vi "gaussmeter_setup.vi"(0 "VISA resource name Gaussmeter":refnum<visa-resource-name>, 1 "Switch Gaussmeter":bool, 2 "Gaussmeter Number":u8, 3 "Moving Gaussmeter":bool, 4 "x Gaussmeter":dbl, 5 "error in (no error)":errorcluster, 7 "y Gaussmeter":dbl, 9 "z Gaussmeter":dbl) -> (6 "Probe Type":u16(ring)=40 items=["High Sensitivity"=40, "High Stability"=41, "Ultra-High Sensitivity"=42, "User Programmable Cable / High Sensitivity Probe"=50, "User Programmable Cable / High Stability Probe"=51, "User Programmable Cable / Ultra-High Sensitivity Probe"=52], 8 "Probe Serial Number":string, 10 "Probe Sensitivity":dbl=0.001 format="%^.3e", 12 "Probe Field\nCompensation On":bool, 13 "Status Gaussmeter":bool, 14 "Gaussmeter VISA resource name out":refnum<visa-resource-name>, 15 "Field Range":u16(ring)=1 items=["1 - Lowest"=1, "2"=2, "3"=3, "4 - Highest"=4], 16 "Field Units":u16(ring)=1 items=["Gauss"=1, "Tesla"=2, "Oersted"=3, "Amp/Meter"=4], 17 "Auto Range On":bool, 18 "Text Output":string, 19 "error out":errorcluster)   [LabVIEW 2016]
uses:
  <instrlib>/Lake Shore 425/Lake Shore 425.lvlib
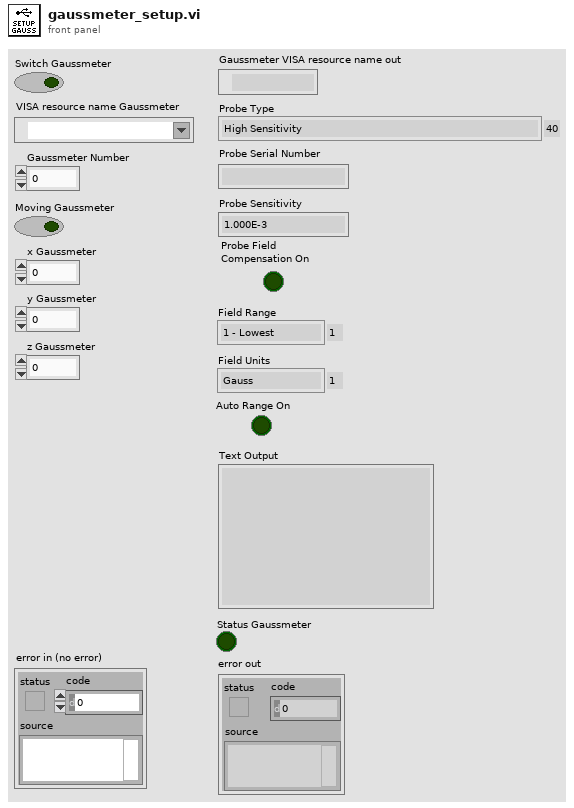
[diagram p1: front panel]
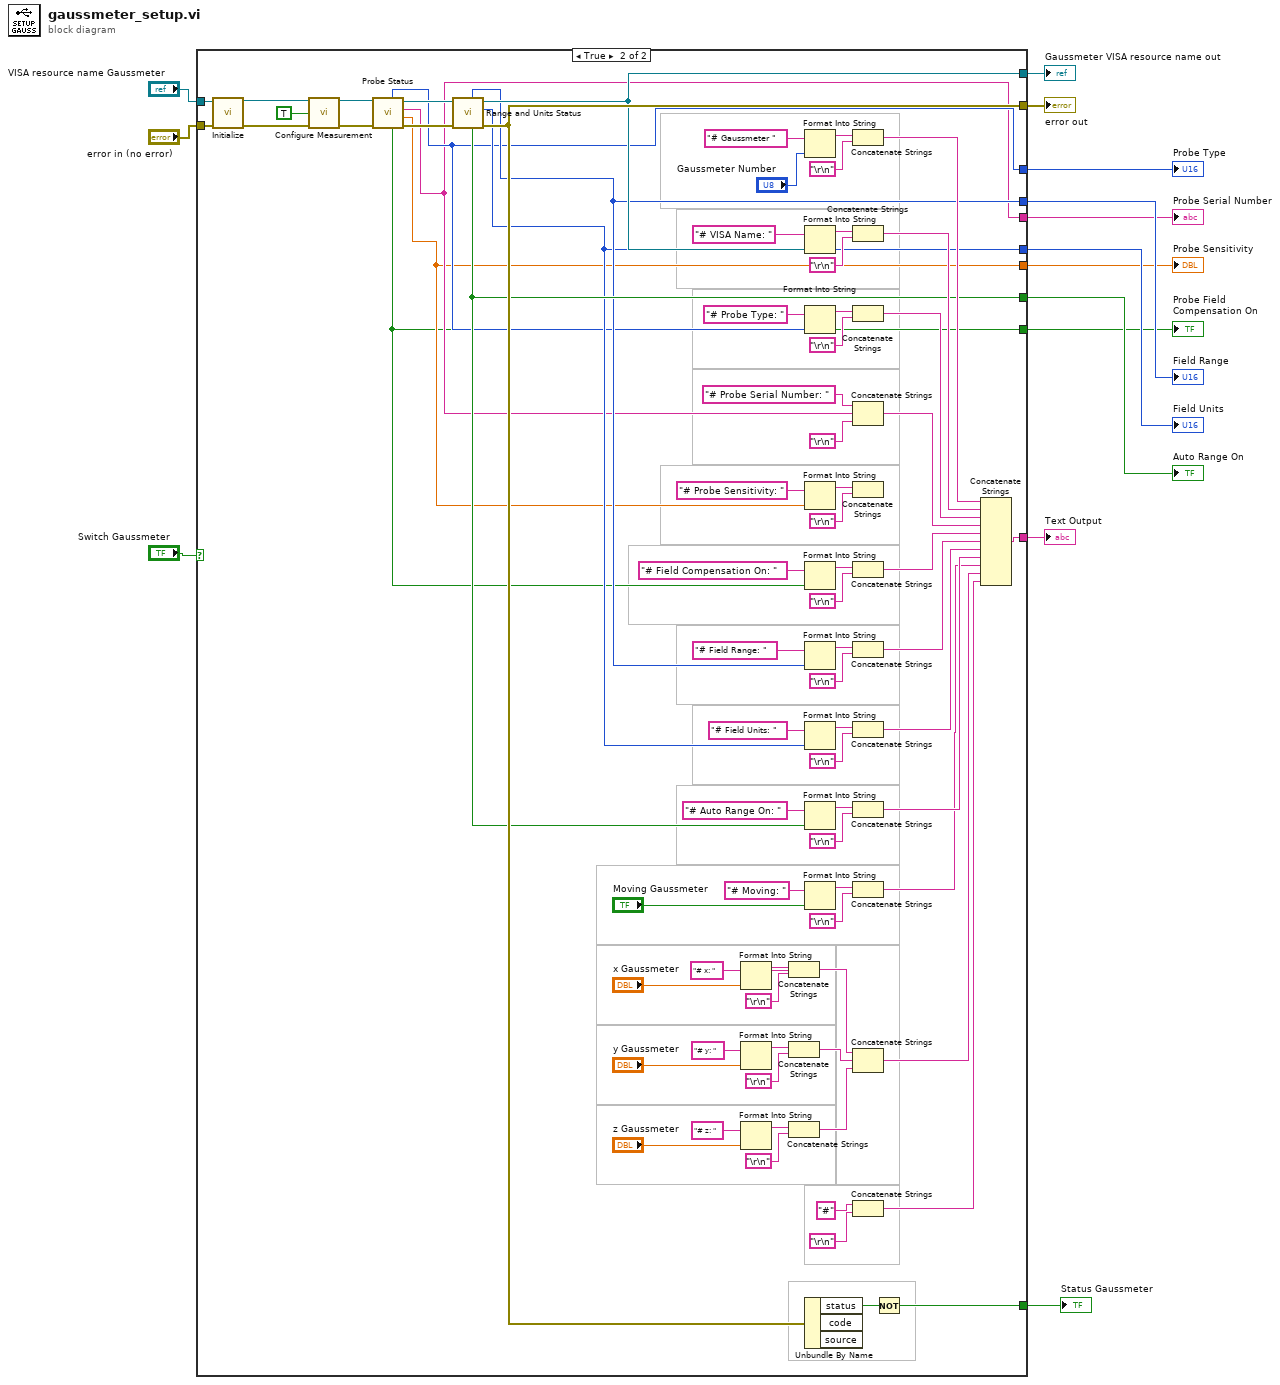
[diagram p0: block diagram]
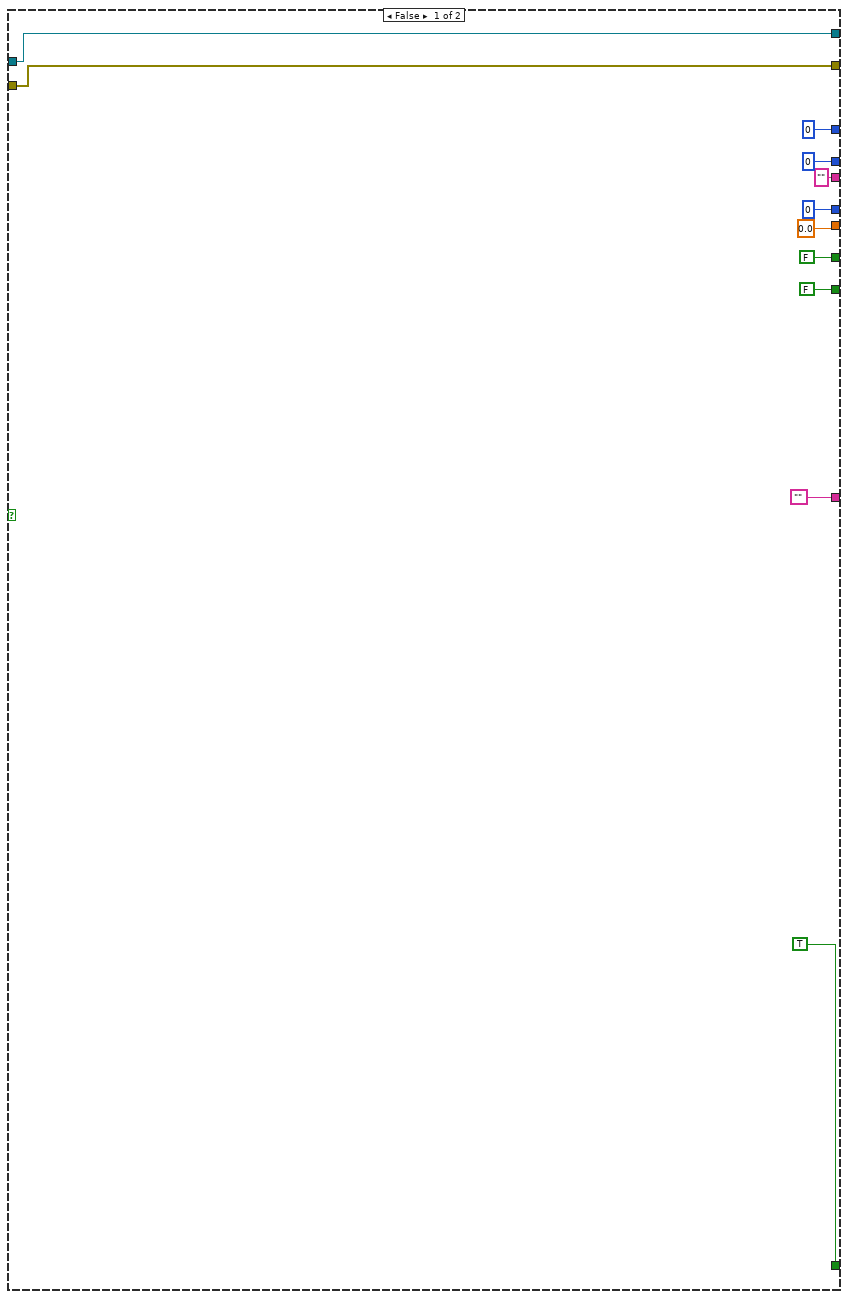
[diagram p2: hidden frame]
diagram:
  n1 = case shown="True" "Switch Gaussmeter" {
    tunnel: "VISA resource name Gaussmeter" -> [w25 w105]
    tunnel: "error in (no error)" -> [w24 w104]
    tunnel: ["" w63] -> w12
    tunnel: [TRUE w61] -> w11
    tunnel: [w24 w60] -> w10
    tunnel: [w25 w59] -> w9
    tunnel: [FALSE ("Auto Range On") w58] -> w7
    tunnel: [u16 0 ("Field Range") w57] -> w6
    tunnel: [u16 0 ("Field Units") w56] -> w5
    tunnel: [u16 0 ("Probe Type") w55] -> w4
    tunnel: ["" ("Probe Serial Number") w54] -> w3
    tunnel: [0.0 ("Probe Sensitivity") w53] -> w2
    tunnel: [FALSE ("Probe Field \nCompensation On") w52] -> w1
    frame False {
    }
    frame True {
      n2 = call <instrlib>:"Initialize.vi"("error in (no error)"=w104, "VISA resource name"=w105) -> ("error out"=w27:errorcluster, "VISA resource name out"=w28:refnum<visa-resource-name>)  [unwired: 8 in]
      n3 = call <instrlib>:"Configure Measurement.vi"("VISA resource name"=w28, "Filter (F: Off)"=TRUE, "error in (no error)"=w27) -> ("VISA resource name out"=w30:refnum<visa-resource-name>, "error out"=w29:errorcluster)  [unwired: 11 in]
      n4 = call <instrlib>:"Probe Status.vi"("error in (no error)"=w29, "VISA resource name"=w30) -> ("error out"=w102:errorcluster, "Probe Sensitivity"=w53:dbl, "Probe Serial Number"=w54:string, "VISA resource name out"=w103:refnum<visa-resource-name>, "Probe Field \nCompensation On"=w52:bool, "Probe Type"=w55:u16)  [unwired: 4 in]
      n5 = call <instrlib>:"Range and Units Status.vi"("error in (no error)"=w102, "VISA resource name"=w103) -> ("error out"=w60:errorcluster, "Field Units"=w56:u16, "VISA resource name out"=w59:refnum<visa-resource-name>, "Auto Range On"=w58:bool, "Field Range"=w57:u16)  [unwired: 5 in]
      n6 = Format Into String(initial string="# x: ", "x Gaussmeter") -> (resulting string=w50:string)  [unwired: 2 in, 1 out]
      n7 = Format Into String(initial string="# y: ", "y Gaussmeter") -> (resulting string=w47:string)  [unwired: 2 in, 1 out]
      n8 = Format Into String(initial string="# z: ", "z Gaussmeter") -> (resulting string=w41:string)  [unwired: 2 in, 1 out]
      n9 = Concatenate Strings(w50, "\r\n") -> (w39:string)
      n10 = Concatenate Strings(w47, "\r\n") -> (w38:string)
      n11 = Concatenate Strings(w41, "\r\n") -> (w37:string)
      n12 = Format Into String(initial string="# Gaussmeter ", "Gaussmeter Number") -> (resulting string=w99:string)  [unwired: 2 in, 1 out]
      n13 = Format Into String(initial string="# VISA Name: ", w59) -> (resulting string=w87:string)  [unwired: 2 in, 1 out]
      n14 = Format Into String(initial string="# Probe Type: ", w55) -> (resulting string=w88:string)  [unwired: 2 in, 1 out]
      n15 = Format Into String(initial string="# Probe Sensitivity: ", w53) -> (resulting string=w89:string)  [unwired: 2 in, 1 out]
      n16 = Format Into String(initial string="# Field Compensation On: ", w52) -> (resulting string=w86:string)  [unwired: 2 in, 1 out]
      n17 = Format Into String(initial string="# Field Range: ", w57) -> (resulting string=w84:string)  [unwired: 2 in, 1 out]
      n18 = Format Into String(initial string="# Field Units: ", w56) -> (resulting string=w82:string)  [unwired: 2 in, 1 out]
      n19 = Format Into String(initial string="# Auto Range On: ", w58) -> (resulting string=w79:string)  [unwired: 2 in, 1 out]
      n20 = Format Into String(initial string="# Moving: ", "Moving Gaussmeter") -> (resulting string=w44:string)  [unwired: 2 in, 1 out]
      n21 = Unbundle By Name(w60) -> ("status"=w62:bool)  [unwired: 2 out]
      n22 = Concatenate Strings(w99, "\r\n") -> (w74:string)
      n23 = Concatenate Strings(w87, "\r\n") -> (w73:string)
      n24 = Concatenate Strings(w88, "\r\n") -> (w72:string)
      n25 = Concatenate Strings("# Probe Serial Number: ", w54, "\r\n") -> (w71:string)
      n26 = Concatenate Strings(w89, "\r\n") -> ()  [unwired: 1 out]
      n27 = Concatenate Strings(w86, "\r\n") -> (w70:string)
      n28 = Concatenate Strings(w84, "\r\n") -> (w69:string)
      n29 = Concatenate Strings(w82, "\r\n") -> (w68:string)
      n30 = Concatenate Strings(w79, "\r\n") -> (w67:string)
      n31 = Concatenate Strings(w44, "\r\n") -> (w35:string)
      n32 = Concatenate Strings(w39, w38, w37) -> (w36:string)
      n33 = Concatenate Strings("#", "\r\n") -> (w64:string)
      n34 = Not(x=w62) -> (.not. x?=w61:bool)
      n35 = Concatenate Strings(w74, w73, w72, w71, w70, w69, w68, w67, w35, w36, w64) -> (w63:string)
    }
  }
  "Text Output" <- w12
  "Status Gaussmeter" <- w11
  "error out" <- w10
  "Gaussmeter VISA resource name out" <- w9
  "Auto Range On" <- w7
  "Field Units" <- w5
  "Field Range" <- w6
  "Probe Type" <- w4
  "Probe Serial Number" <- w3
  "Probe Sensitivity" <- w2
  "Probe Field\nCompensation On" <- w1
